vi "maximini_XYlist.vi"() -> ()   [LabVIEW 2013]
uses:
  <vilib>/Analysis/Matrix/Datatypes/RealMatrix.ctl
  <vilib>/Analysis/Matrix/NI_Matrix.lvlib
panel:
  out "maxi Y":dbl
  out "maxi X":dbl
  out "mini Y":dbl
  out "mini X":dbl
  in  "stored XY":T1
  in  "LY":dbl
  in  "LX":dbl
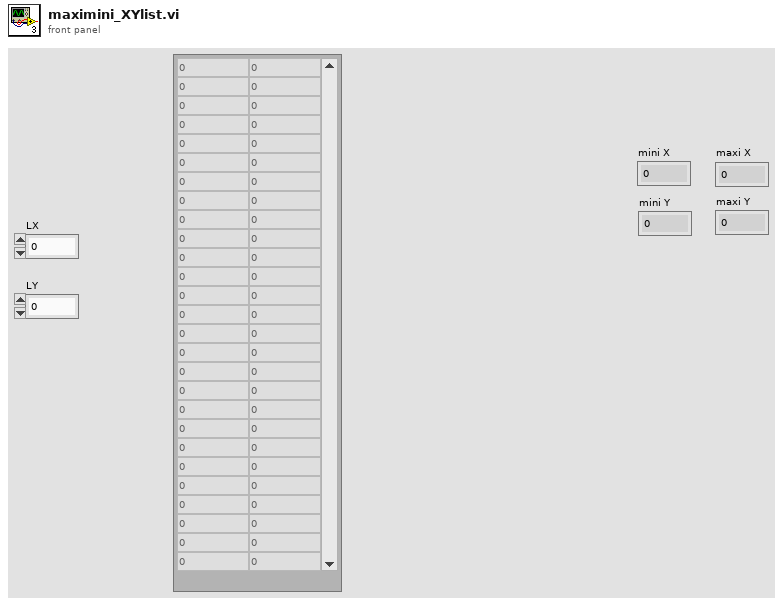
[diagram p1: front panel]
types:
  T1 = typedef "NI_Matrix.lvlib/RealMatrix.ctl" = dbl[][]
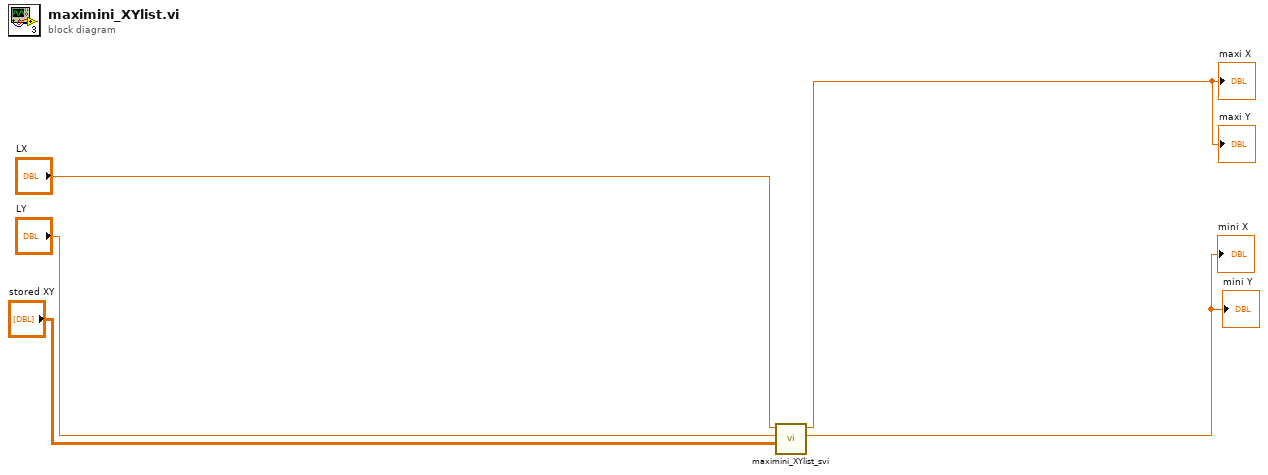
[diagram p0: block diagram]
diagram:
  n1 = call "maximini_XYlist_svi.vi"("stored XY"="stored XY", "LY"="LY", "LX"="LX") -> ("Numérique 2"=→"mini X" →"mini Y":dbl, "Numérique"=→"maxi X" →"maxi Y":dbl)  [unwired: 7 in]
